vi "HELP.vi"(8 "error in (no error)":errorcluster, 11 "Instrument in":refnum<class "Instrument.lvclass">) -> (0 "error out":errorcluster, 2 "Commands":string[](array[string]), 3 "Instrument out":refnum<class "Instrument.lvclass">)   [LabVIEW 2020, in "Instrument.lvclass"]
uses:
  Instrument.lvclass
  Typedefs/Instrument.Commands--Enum.ctl
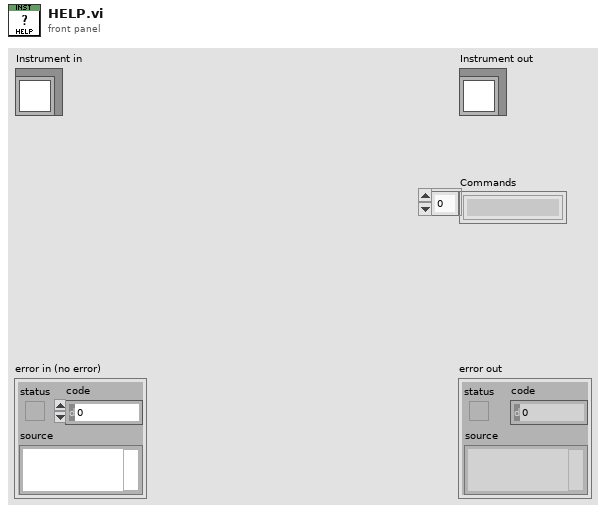
[diagram p1: front panel]
types:
  T1 = typedef "Instrument.lvclass/Instrument.Commands--Enum.ctl" = enum16{"HELP", "ACK", "getAll"}
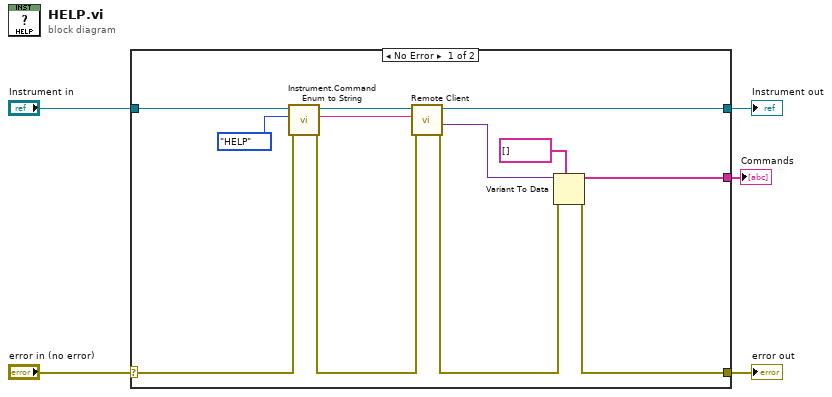
[diagram p0: block diagram]
diagram:
  n1 = case shown="No Error" "error in (no error)" {
    selector: "error in (no error)" -> [w7 w19]
    tunnel: [w14 w19] -> w4
    tunnel: [w17 w18] -> w2
    tunnel: "Instrument in" -> [w11 w18]
    tunnel: [w13 _] -> w1
    frame No Error {
      n2 = call "Instrument.Command Enum to String.vi"("error in (no error)"=w7, "Commands"=Instrument.Commands--Enum."HELP", "Instrument in"=w11) -> ("error out"=w6:errorcluster, "Command"=w8:string, "Instrument out"=w10:refnum<class "Instrument.lvclass">)  [unwired: 5 in, 1 out]
      n3 = call "Remote Client.vi"("error in (no error)"=w6, "Command"=w8, "Instrument in"=w10) -> ("error out"=w15:errorcluster, "Data out"=w16:variant, "Instrument out"=w17:refnum<class "Instrument.lvclass">)  [unwired: 5 in, 1 out]
      n4 = Variant To Data(error in=w15, type=string[] [] ("Commands"), Variant=w16) -> (data=w13:string[], error out=w14:errorcluster)
    }
    frame Error {
    }
  }
  "error out" <- w4
  "Instrument out" <- w2
  "Commands" <- w1
